vi "File2.List Files and SubFolders.vi"(8 "error in (no error)":errorcluster, 11 "Folder":path) -> (0 "error out":errorcluster, 2 "Folders":path[](array[path]), 3 "Files":path[](array[path]))   [LabVIEW 2024]
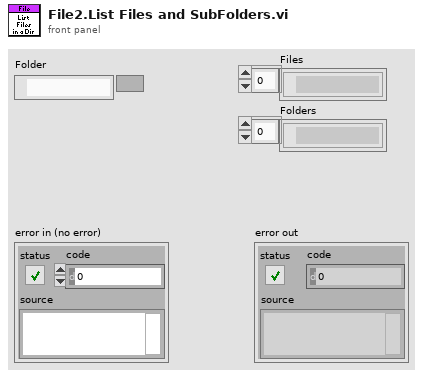
[diagram p1: front panel]
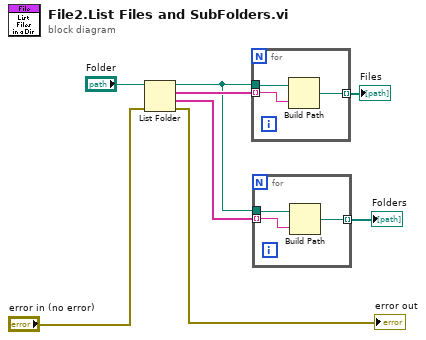
[diagram p0: block diagram]
diagram:
  n1 = List Folder(path="Folder", error in="error in (no error)") -> (path out=w7:path, filenames=w8:string[], folder names=w6:string[], error out=→"error out":errorcluster)  [unwired: 2 in]
  n2 = for {
    tunnel: w7 -> [w11]
    tunnel: w8 -> [w10] mode=indexing
    tunnel: [w9] -> w5 mode=indexing
    n3 = Build Path(base path=w11, name or relative path=w10) -> (appended path=w9:path)
  }
  "Files" <- w5
  n4 = for {
    tunnel: w7 -> [w14]
    tunnel: w6 -> [w13] mode=indexing
    tunnel: [w12] -> w4 mode=indexing
    n5 = Build Path(base path=w14, name or relative path=w13) -> (appended path=w12:path)
  }
  "Folders" <- w4
